vi "Auton Up or Down.vi"(9 "Current Position (deg)":dbl, 11 "Current Setpoint (deg)":dbl) -> (3 "Moving UP?":bool)   [LabVIEW 2011]
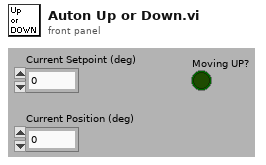
[diagram p1: front panel]
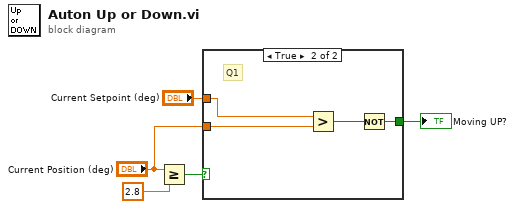
[diagram p0: block diagram]
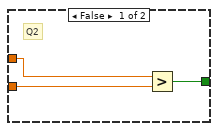
[diagram p2: hidden frame]
diagram:
  n1 = Greater Or Equal?(x="Current Position (deg)", y=2.8) -> (x >= y?=w4:bool)
  n2 = case shown="True" w4 {
    tunnel: "Current Setpoint (deg)" -> [w8 w12]
    tunnel: [w6 w9] -> w2
    tunnel: "Current Position (deg)" -> [w7 w11]
    frame False {
      # "Q2"
      n3 = Greater?(x=w8, y=w7) -> (0:w6:bool)
    }
    frame True {
      # "Q1"
      n4 = Greater?(x=w12, y=w11) -> (0:w10:bool)
      n5 = Not(x=w10) -> (.not. x?=w9:bool)
    }
  }
  "Moving UP?" <- w2
